vi "principal.vi"() -> ()   [LabVIEW 2018]
uses:
  Global vars.vi
panel:
  in  "stop":bool
  out "L3":bool
  out "L2":bool
  out "L1":bool
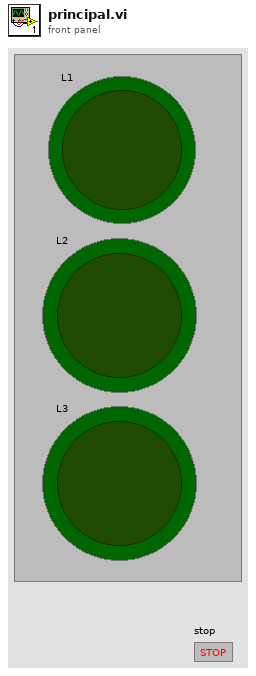
[diagram p1: front panel]
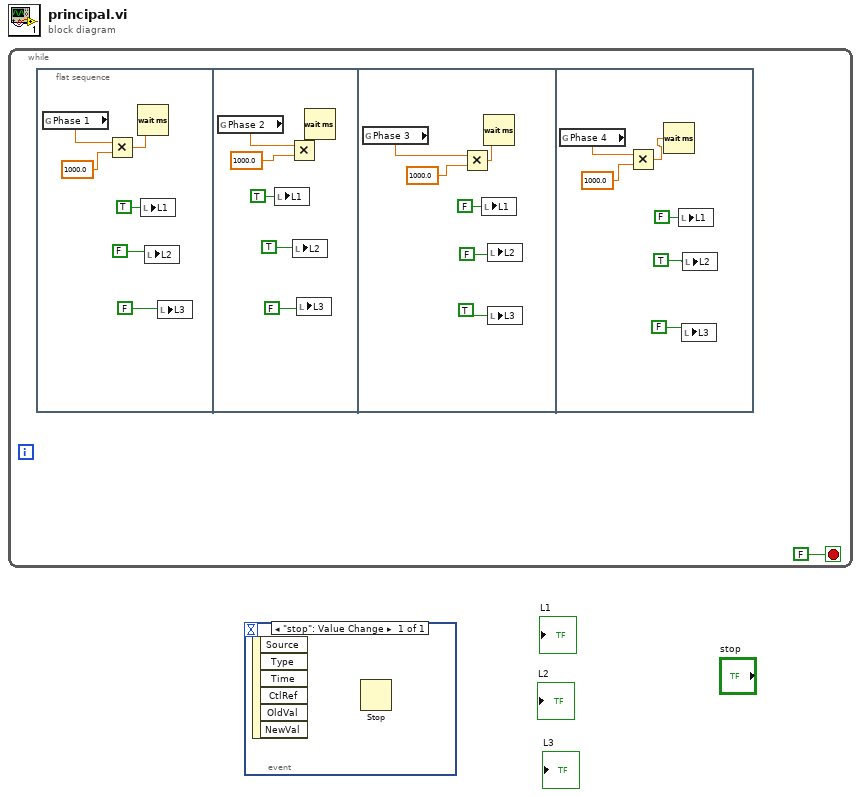
[diagram p0: block diagram]
diagram:
  n1 = while {
    stop <- FALSE stop-if-true
    n2 = flat-sequence {
      frame #0 {
        n3 = global read "Global vars.vi" "Phase 1"() -> (w4:dbl)
        n4 = Multiply(x=w4, y=1000.0) -> (x*y=w3:dbl)
        n5 = Wait (ms)(milliseconds to wait=w3) -> ()  [unwired: 1 out]
        n6 = local write "L1"(TRUE ("L1")) -> ()
        n7 = local write "L2"(FALSE ("L1")) -> ()
        n8 = local write "L3"(FALSE ("L1")) -> ()
      }
      frame #1 {
        n9 = global read "Global vars.vi" "Phase 2"() -> (w9:dbl)
        n10 = local write "L1"(TRUE ("L1")) -> ()
        n11 = Multiply(x=w9, y=1000.0) -> (x*y=w8:dbl)
        n12 = local write "L2"(TRUE ("L1")) -> ()
        n13 = local write "L3"(FALSE ("L1")) -> ()
        n14 = Wait (ms)(milliseconds to wait=w8) -> ()  [unwired: 1 out]
      }
      frame #2 {
        n15 = global read "Global vars.vi" "Phase 3"() -> (w14:dbl)
        n16 = Multiply(x=w14, y=1000.0) -> (x*y=w15:dbl)
        n17 = local write "L1"(FALSE ("L1")) -> ()
        n18 = Wait (ms)(milliseconds to wait=w15) -> ()  [unwired: 1 out]
        n19 = local write "L2"(FALSE ("L1")) -> ()
        n20 = local write "L3"(TRUE ("L1")) -> ()
      }
      frame #3 {
        n21 = global read "Global vars.vi" "Phase 4"() -> (w21:dbl)
        n22 = Multiply(x=w21, y=1000.0) -> (x*y=w20:dbl)
        n23 = Wait (ms)(milliseconds to wait=w20) -> ()  [unwired: 1 out]
        n24 = local write "L1"(FALSE ("L1")) -> ()
        n25 = local write "L3"(FALSE ("L1")) -> ()
        n26 = local write "L2"(TRUE ("L1")) -> ()
      }
    }
  }
  n27 = event shown="[0] \"stop\": Value Change" {
    selector: _ -> [_]
    dyn-events: _ -> [_]
    timeout: _ -> [_]
    event "stop": Value Change {
      n28 = event-data() -> ()  [unwired: 1 in, 6 out]
      n29 = Stop() -> ()  [unwired: 1 in]
    }
  }
